vi "Process buy.vi"(8 "error in (no error)":errorcluster, 10 "Compra":bool, 11 "USD Actor in":refnum<class "USD Actor.lvclass">) -> (0 "error out":errorcluster, 3 "USD Actor out":refnum<class "USD Actor.lvclass">)   [LabVIEW 2020, in "USD Actor.lvlib" / "USD Actor.lvclass"]
uses:
  USD Actor.lvclass
  C:/Program Files/National Instruments/LabVIEW 2020/vi.lib/ActorFramework/Actor/Actor.lvclass
  Soda Actor/Soda Actor.lvclass
  Soda Actor/Soda Actor.lvclass/Soda Actor.ctl
  USD Actor.lvclass/USD Actor.ctl
  <vilib>/ActorFramework/Actor/Actor.lvclass/Actor.ctl
  UI Actor Messages/credit update Msg/credit update Msg.lvclass/credit update Msg.ctl
  <vilib>/ActorFramework/Message Enqueuer/Message Enqueuer.lvclass/Message Enqueuer.ctl
  <vilib>/ActorFramework/Message Enqueuer/Enqueue.vi
  UI Actor Messages/credit update Msg/credit update Msg.lvclass
  C:/Program Files/National Instruments/LabVIEW 2020/vi.lib/ActorFramework/Message/Message.lvclass
  <vilib>/Utility/config.llb/Read Key (Double).vi
  <vilib>/ActorFramework/Message Priority Queue/Priority Enqueue.vi
  <vilib>/ActorFramework/Actor/Actor.lvclass
  <vilib>/Utility/config.llb/NI_LVConfig.lvlib
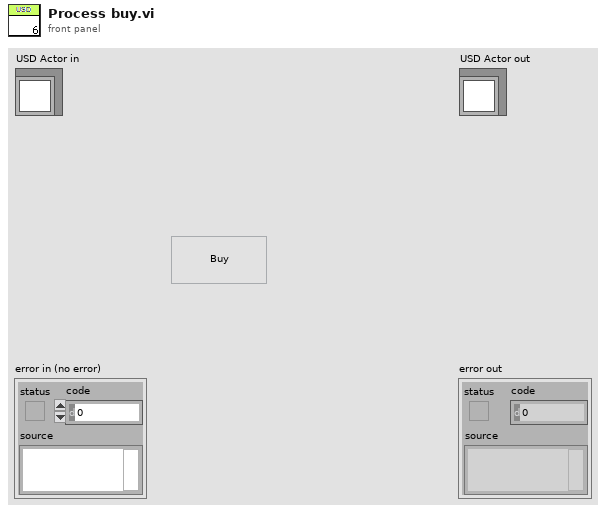
[diagram p1: front panel]
types:
  T1 = typedef "NI_LVConfig.lvlib/Config Data RefNum.ctl" = refnum<k1>
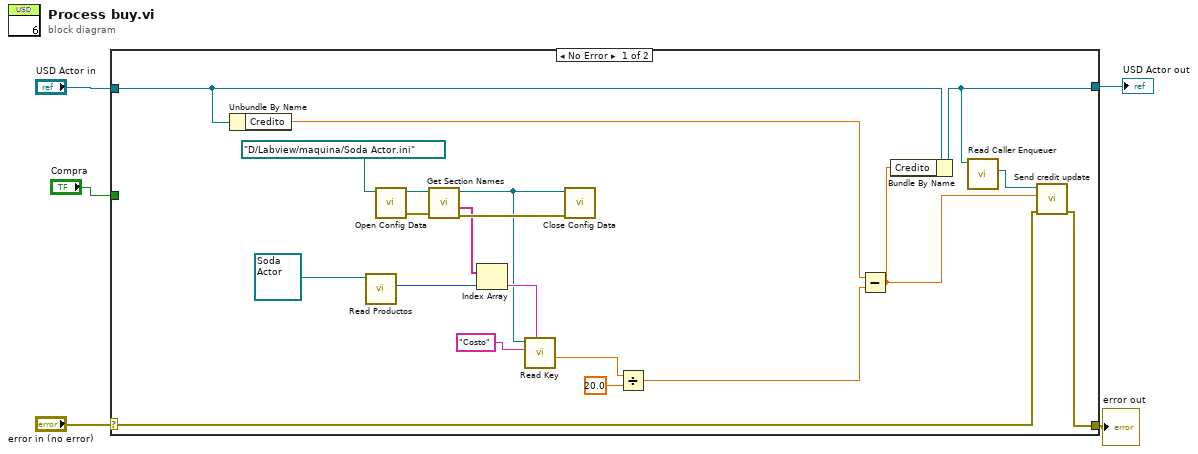
[diagram p0: block diagram]
diagram:
  n1 = case shown="No Error" "error in (no error)" {
    selector: "error in (no error)" -> [w23 w27]
    tunnel: [w22 w27] -> w4
    tunnel: [w25 w26] -> w2
    tunnel: "USD Actor in" -> [w8 w26]
    tunnel: "Compra" -> [_ _]
    frame No Error {
      n2 = Unbundle By Name(w8) -> ("Credito"=w17:dbl)
      n3 = call "Read Productos.vi"("Soda Actor in"=refnum<class "Soda Actor.lvclass"> refnum ("Soda Actor.lvlib:Soda Actor.lvclass")) -> ("Productos"=w7:i32)  [unwired: 8 in, 2 out]
      n4 = call <vilib>:"Open Config Data.vi"("configuration file path"=path "D:/Labview/maquina/Soda Actor.ini") -> ("error out"=w21:errorcluster, "refnum"=w20:T1)  [unwired: 8 in, 1 out]
      n5 = call <vilib>:"Get Section Names.vi"("error in (no error)"=w21, "refnum"=w20) -> ("error out"=w19:errorcluster, "section names"=w15:string[], "refnum out"=w12:T1)  [unwired: 7 in]
      n6 = Index Array(array=w15, index=w7) -> (element=w14:string)
      n7 = call-poly <vilib>:"Read Key.vi"("section"=w14, "key"="Costo", "refnum"=w12) -> ("value"=w11:dbl)  [unwired: 5 in, 3 out]
      n8 = call <vilib>:"Close Config Data.vi"("error in (no error)"=w19, "refnum"=w12) -> ()  [unwired: 8 in, 2 out]
      n9 = Divide(x=w11, y=20.0) -> (x/y=w9:dbl)
      n10 = Subtract(x=w17, y=w9) -> (x-y=w16:dbl)
      n11 = Bundle By Name(cluster=w8, "Credito"=w16) -> (w25:refnum<class "USD Actor.lvclass">)
      n12 = call <vilib>:"Read Caller Enqueuer.vi"("Actor"=w25) -> ("Caller Enqueuer"=w24:refnum<class "Message Enqueuer.lvclass">)  [unwired: 10 in]
      n13 = call "Send credit update.vi"("error in (no error)"=w23, "credito"=w16, "Message Enqueuer"=w24) -> ("error out"=w22:errorcluster)  [unwired: 7 in, 1 out]
    }
    frame Error {
    }
  }
  "error out" <- w4
  "USD Actor out" <- w2
